vi "Magnitudes Measurement.vi"(8 "error in":errorcluster, 11 "wfm":waveform(dbl)) -> (0 "error out":errorcluster, 2 "Magnitude RMS":cluster{dbl[], "magnitude":dbl[]}, 3 "Magnitude Peak":cluster{dbl[], dbl[]})   [LabVIEW 2024, in "NIScopeFrequencyDomain.lvlib"]
uses:
  NIScopeFrequencyDomain.lvlib
  <vilib>/measure/maspectr.llb/FFT Spectrum (Mag-Phase) for 1 Chan.vi
  <vilib>/measure/NI_MAPro.lvlib
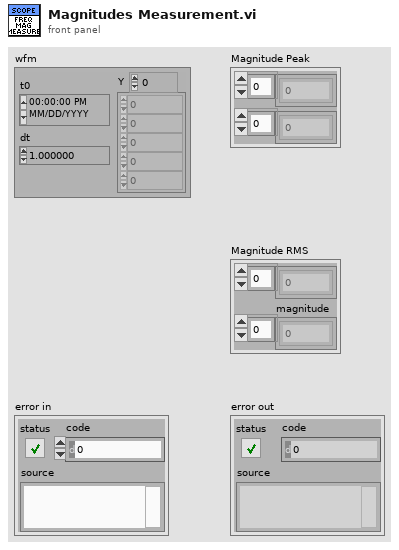
[diagram p1: front panel]
types:
  T1 = cluster{"dB On (F)":bool, "unwrap phase (F)":bool, "convert to degree (F)":bool}
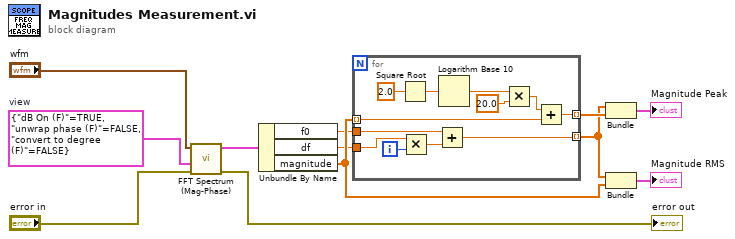
[diagram p0: block diagram]
diagram:
  w1 = T1 {"dB On (F)"=TRUE, "unwrap phase (F)"=FALSE, "convert to degree (F)"=FALSE}  # view
  n1 = call-poly <vilib>:"FFT Spectrum (Mag-Phase).vi"("error in (no error)"="error in", "view"=w1, "time signal"="wfm") -> ("error out"=→"error out":errorcluster, "magnitude"=w4:cluster{"f0":dbl, "df":dbl, "magnitude":dbl[]})  [unwired: 4 in, 3 out]
  n2 = Unbundle By Name(w4) -> ("f0"=w3:dbl, "df"=w5:dbl, "magnitude"=w6:dbl[])
  n3 = for {
    tunnel: w3 -> [w24]
    tunnel: w5 -> [w21]
    tunnel: [w20] -> w7 mode=indexing
    tunnel: w6 -> [w18] mode=indexing
    tunnel: [w13] -> w8 mode=indexing
    i -> [w23]
    n4 = Square Root(x=2.0) -> (sqrt(x)=w17:dbl)
    n5 = Multiply(x=w21, y=w23) -> (x*y=w22:dbl)
    n6 = Add(x=w24, y=w22) -> (x+y=w20:dbl)
    n7 = Logarithm Base 10(1:w17) -> (0:w16:dbl)
    n8 = Multiply(x=w16, y=20.0) -> (x*y=w14:dbl)
    n9 = Add(x=w14, y=w18) -> (x+y=w13:dbl)
  }
  n10 = Bundle(w7, w8) -> (→"Magnitude Peak":cluster{dbl[], dbl[]})  [unwired: 1 in]
  n11 = Bundle(w7, "magnitude"=w6) -> (→"Magnitude RMS":cluster{dbl[], "magnitude":dbl[]})  [unwired: 1 in]
